vi "getChannelStates.vi"(8 "error in (no error)":errorcluster, 11 "rf in":refnum<class "rf.lvclass">) -> (0 "error out":errorcluster, 2 "statesValues":string[](array[string]), 3 "rf out":refnum<class "rf.lvclass">)   [LabVIEW 2011, in "Tools.lvlib" / "Scripting.lvlib" / "rf.lvclass"]
uses:
  rf.lvclass
  DatabaseHelpers/Database Objects/Channel/RfOutputChannel/RfOutputChannel.lvclass
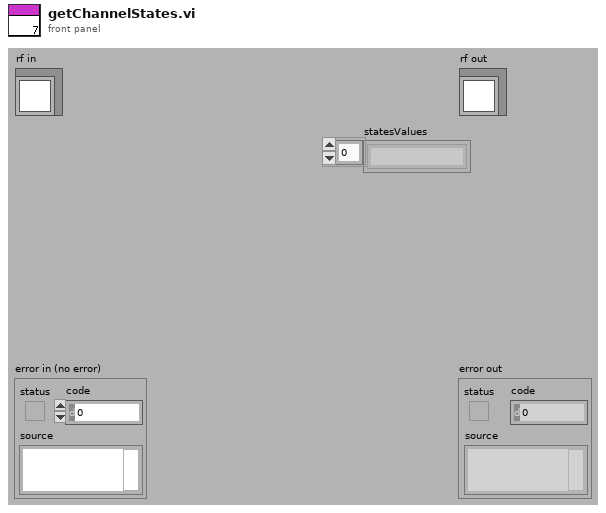
[diagram p1: front panel]
types:
  T1 = cluster{"state_name":string, "value":cluster{"frequency":string, "amplitude":string, "phase":string}}[]
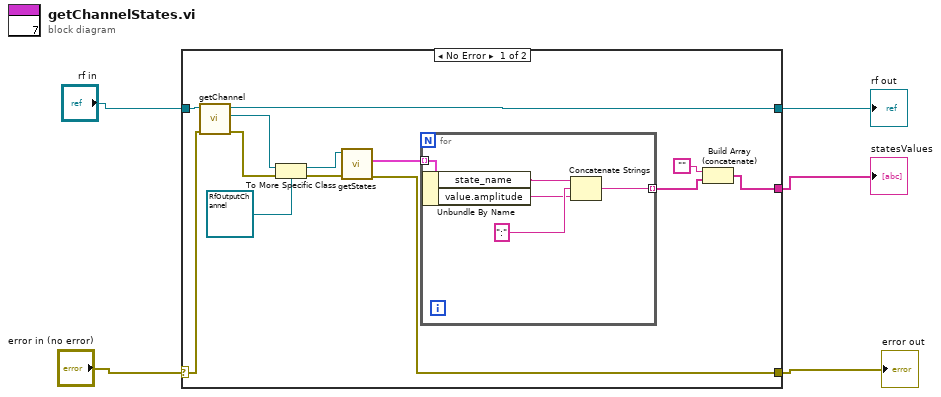
[diagram p0: block diagram]
diagram:
  n1 = case shown="No Error" "error in (no error)" {
    selector: "error in (no error)" -> [w13 w25]
    tunnel: [w12 w25] -> w2
    tunnel: [w14 w24] -> w3
    tunnel: "rf in" -> [w15 w24]
    tunnel: [w17 _] -> w1
    frame No Error {
      n2 = call-dynamic "getChannel.vi"("error in (no error)"=w13, "ScriptEvent.lvclass in"=w15) -> ("error out"=w9:errorcluster, "Channel.lvclass"=w8:refnum<class "Channel.lvclass">, "ScriptEvent.lvclass out"=w14:refnum<class "rf.lvclass">)  [unwired: 7 in]
      n3 = To More Specific Class(target class=refnum<class "RfOutputChannel.lvclass"> refnum ("Tools.lvlib:DatabaseHelpers.lvlib:RfOutputChannel.lvclass"), reference=w8, error in=w9) -> (specific class reference=w7:refnum<class "RfOutputChannel.lvclass">, error out=w11:errorcluster)
      n4 = call "getStates.vi"("error in (no error)"=w11, "RfOutputChannel in"=w7) -> ("error out"=w12:errorcluster, "states"=w6:T1)  [unwired: 7 in, 1 out]
      n5 = for {
        tunnel: w6 -> [w23] mode=indexing
        tunnel: [w19] -> w18 mode=indexing
        n6 = Unbundle By Name(w23) -> ("state_name"=w22:string, "value.amplitude"=w20:string)
        n7 = Concatenate Strings(w22, ":", w20) -> (w19:string)
      }
      n8 = Build Array (concatenate)("", w18) -> (w17:string[])
    }
    frame Error {
    }
  }
  "error out" <- w2
  "rf out" <- w3
  "statesValues" <- w1
